vi "Array Element Product (1D x 1D).vi"(1 "array a":dbl[](array[numeric]), 4 "array b":dbl[](array[numeric])) -> (15 "a * b":dbl[](array[numeric]))   [LabVIEW 2014]
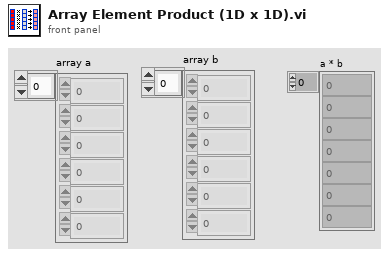
[diagram p1: front panel]
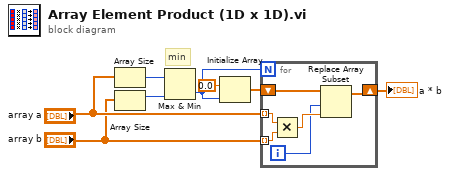
[diagram p0: block diagram]
diagram:
  # "min"
  n1 = Array Size(array="array a") -> (size(s)=w6:i32)
  n2 = Array Size(array="array b") -> (size(s)=w5:i32)
  n3 = Max & Min(x=w6, y=w5) -> (min(x,y)=w4:i32)  [unwired: 1 out]
  n4 = Initialize Array(0.0 ("element"), w4) -> (w2:dbl[])
  n5 = for {
    N: w4 -> [_]
    tunnel: "array a" -> [w13] mode=indexing
    shift-right: [w11] -> w1
    shift-left: w2 -> [w12]
    tunnel: "array b" -> [w14] mode=indexing
    i -> [w9]
    n6 = Multiply(x=w13, y=w14) -> (x*y=w10:dbl)
    n7 = Replace Array Subset(array=w12, new element=w10, index=w9) -> (w11:dbl[])
  }
  "a * b" <- w1
